vi "To Table Test.vi"() -> ()   [LabVIEW 2013, in "User Control Module Test.lvlib"]
uses:
  User Control Module Test.lvlib
  <vilib>/NI/Module Execution Interface/Engine Configuration/engine configuration.lvclass
  <vilib>/NI/Tag Bus/tag/tag descriptor.lvclass
  editor node/user control module editor.lvclass
  <vilib>/NI/Tag Bus/tag/tag descriptor.lvclass/tag descriptor.ctl
  <vilib>/NI/Configuration Framework/serializable configuration/NISE_CEF_serializable configuration.lvclass/NISE_CEF_serializable configuration.ctl
  <vilib>/Utility/LVClass/Get LV Class Name.vi
  <vilib>/NI/Configuration Framework/error generator/NISE_error generator.vi
  <vilib>/NI/Configuration Framework/serializable configuration/NISE_CEF_serializable configuration.lvclass
panel:
  out "error out":errorcluster
  out "table":string[][](array[string])
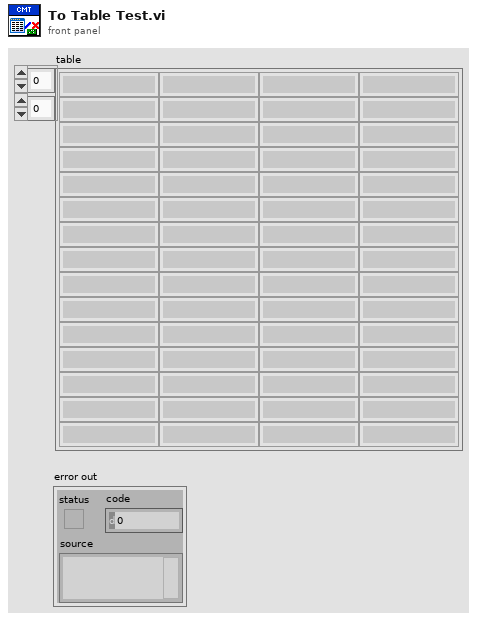
[diagram p1: front panel]
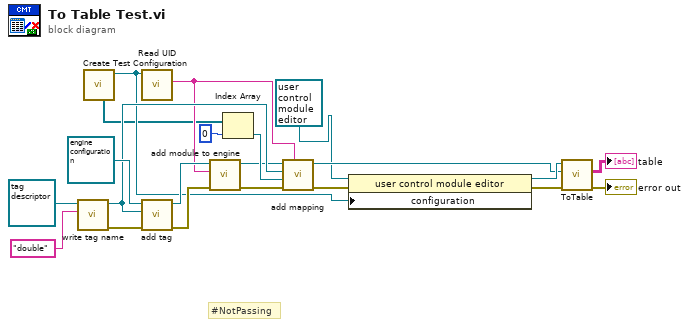
[diagram p0: block diagram]
diagram:
  # "#NotPassing"
  n1 = call <vilib>:"write tag name.vi"("name"="double", "system tag in"=refnum<class "tag descriptor.lvclass"> refnum ("tag descriptor")) -> ("error out"=w6:errorcluster, "system tag out"=w13:refnum<class "tag descriptor.lvclass">)  [unwired: 8 in]
  n2 = call "Create Test Configuration.vi"() -> ("Module"=w5:refnum<class "user control module configuration.lvclass">, "Channels"=w4:refnum<class "TBM channel.lvclass">[])  [unwired: 6 in, 4 out]
  n3 = call <vilib>:"Read UID.vi"("configuration in"=w5) -> ("instance id"=w9:string)  [unwired: 8 in, 2 out]
  n4 = call <vilib>:"add tag.vi"("error in"=w6, "tag descriptor"=w13, "engine configuration in"=refnum<class "engine configuration.lvclass"> refnum ("engine configuration")) -> ("error out"=w7:errorcluster, "engine configuration out"=w11:refnum<class "engine configuration.lvclass">)  [unwired: 7 in]
  n5 = call-dynamic "add module to engine.vi"("error in"=w7, "module ID"=w9, "engine configuration in"=w11) -> ("error out"=w8:errorcluster, "engine configuration out"=w10:refnum<class "engine configuration.lvclass">)  [unwired: 7 in]
  n6 = Index Array(array=w4, index=0) -> (element=w14:refnum<class "TBM channel.lvclass">)
  n7 = call <vilib>:"add mapping.vi"("owner ID"=w9, "error in"=w8, "channel"=w14, "tag descriptor"=w13, "engine configuration"=w10) -> ("error out"=w2:errorcluster, "engine configuration out"=w12:refnum<class "engine configuration.lvclass">)  [unwired: 5 in]
  n8 = property class="user control module editor"(reference=refnum<class "user control module editor.lvclass"> refnum ("user control module editor"), error in=w2, "configuration"=w5) -> (reference out=w21:refnum<class "user control module editor.lvclass">, error out=w3:errorcluster)
  n9 = call-dynamic "ToTable.vi"("error in (no error)"=w3, "variant"=w12, "node in"=w21) -> ("error out"=→"error out":errorcluster, "table"=→"table":string[][])  [unwired: 5 in, 2 out]
